vi "Get Anchor Batch.vi"(2 "Input Array":string[][](array[string]), 3 "Batch size":dbl=3.0) -> (0 "Rest array":string[][](array[string]), 1 "Batch array":string[][](array[string]))   [LabVIEW 2014]
panel:
  # "Batch size = size of rounds.\nSo, if we have anchor IDs 0, 1 & 2 -> batch size = 3"
  # "Returned array with appropriate anchor ID's and distances. Rest array is the original array minus the batch."
  # "VI assumes anchor ID's are ordered"
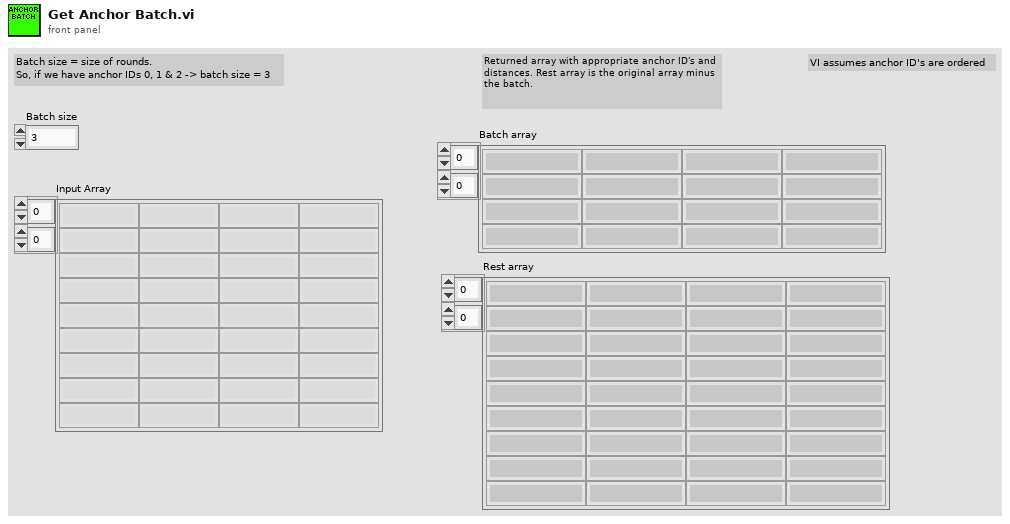
[diagram p1: front panel]
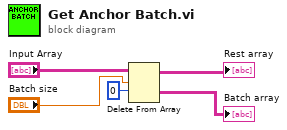
[diagram p0: block diagram]
diagram:
  n1 = Delete From Array(array="Input Array", length="Batch size", index (row)=0) -> (deleted portion=→"Batch array":string[][], array with subset deleted=→"Rest array":string[][])  [unwired: 1 in]
